vi "Convert Assert Event Data to Test Case - Error - Stack Trace.vi"() -> ()   [LabVIEW 2013, in "JUnit Conversion Tests.lvlib"]
uses:
  JUnit Conversion Tests.lvlib
  <vilib>/addons/_JKI Toolkits/Caraya/classes/Test Result/Assert Event Data (Extended).ctl
  JUnit XML/Test Case/Test Case.lvclass/Test Case.ctl
  JUnit XML/Test Case/Read Stack Trace.vi
  <vilib>/addons/_JKI Toolkits/Caraya/classes/Assert/Assert Equal Value_Variant.vi
  JUnit Conversion/JUnit Conversion.lvlib
  <vilib>/addons/_JKI Toolkits/Caraya/classes/Test Result/Test Result.lvclass
  <vilib>/addons/_JKI Toolkits/Caraya/classes/Assert/Assert.lvclass
  <vilib>/addons/_JKI Toolkits/Caraya/classes/Test/Test.lvclass
  JUnit XML/Test Case/Test Case.lvclass
panel:
  out "error out":errorcluster
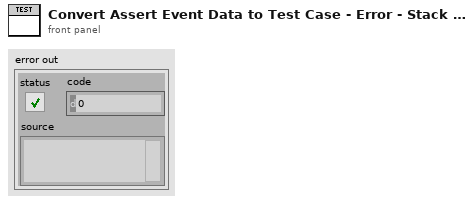
[diagram p1: front panel]
types:
  T1 = typedef "Caraya.lvlib/Test Result.lvclass/Assert Event Data (Extended).ctl" = cluster{"name":string, "passed":bool, "call-chain":string[], "test-error":errorcluster, "timestamp":timestamp, "assert-id":string, "test-id":string, "time":dbl, "message":string, "properties":variant, "measurements":variant, "user-defined":variant}
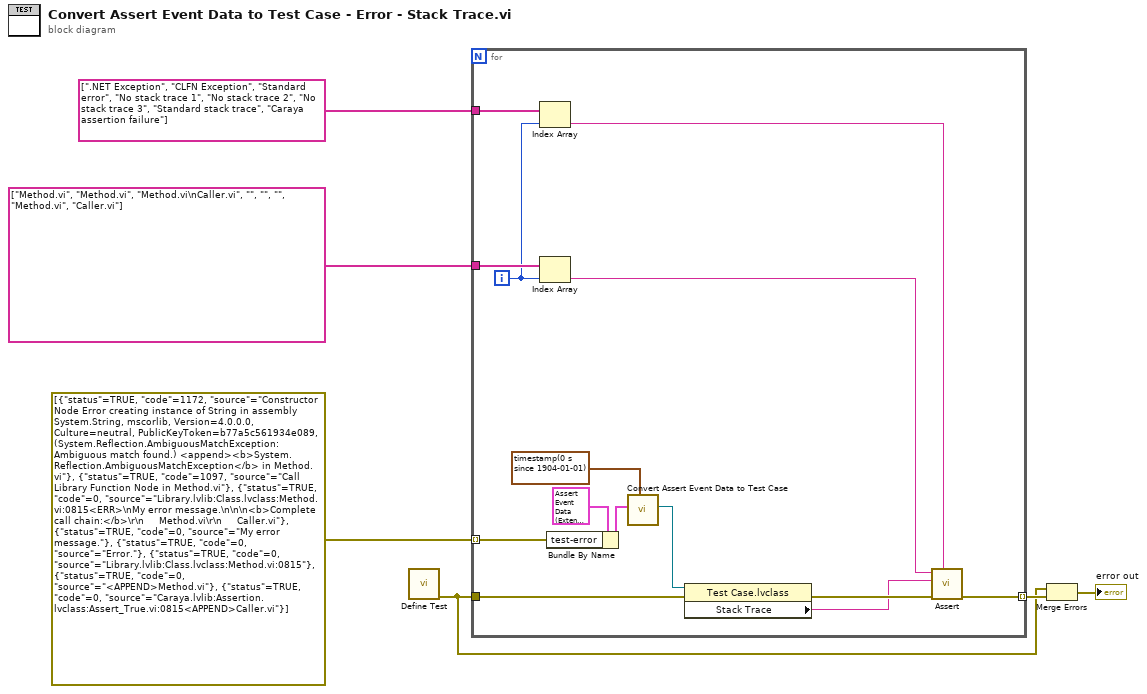
[diagram p0: block diagram]
diagram:
  n1 = call <vilib>:"Define Test.vi"() -> ("error out"=w4:errorcluster)  [unwired: 10 in, 1 out]
  n2 = for {
    tunnel: [w20] -> w6 mode=indexing
    tunnel: w4 -> [w19]
    tunnel: string[] ["Method.vi", "Method.vi", "Method.vi\nCaller.vi", "", "", "", "Method.vi", "Caller.vi"] -> [w13]
    tunnel: errorcluster[] [{"status"=TRUE, "code"=1172, "source"="Constructor Node Error creating instance of String in assembly System.String, mscorlib, Version=4.0.0.0, Culture=neutral, PublicKeyToken=b77a5c561934e089, (System.Reflection.AmbiguousMatchException: Ambiguous match found.) <append><b>System.Reflection.AmbiguousMatchException</b> in Method.vi"}, {"status"=TRUE, "code"=1097, "source"="Call Library Function Node in Method.vi"}, {"status"=TRUE, "code"=0, "source"="Library.lvlib:Class.lvclass:Method.vi:0815<ERR>\nMy error message.\n\n\n<b>Complete call chain:</b>\r\n     Method.vi\r\n     Caller.vi"}, {"status"=TRUE, "code"=0, "source"="My error message."}, {"status"=TRUE, "code"=0, "source"="Error."}, {"status"=TRUE, "code"=0, "source"="Library.lvlib:Class.lvclass:Method.vi:0815"}, {"status"=TRUE, "code"=0, "source"="<APPEND>Method.vi"}, {"status"=TRUE, "code"=0, "source"="Caraya.lvlib:Assertion.lvclass:Assert_True.vi:0815<APPEND>Caller.vi"}] -> [w12] mode=indexing
    tunnel: string[] [".NET Exception", "CLFN Exception", "Standard error", "No stack trace 1", "No stack trace 2", "No stack trace 3", "Standard stack trace", "Caraya assertion failure"] -> [w11]
    i -> [w9]
    n3 = Index Array(array=w11, index=w9) -> (element=w10:string)
    n4 = Index Array(array=w13, index=w9) -> (element=w8:string)
    n5 = Bundle By Name(cluster=T1 {"name"="", "passed"=FALSE, "call-chain"=[], "test-error"={"status"=FALSE, "code"=0, "source"=""}, "timestamp"=timestamp(0 s since 1904-01-01), "assert-id"="", "test-id"="", "time"=-1.0, "message"="", "properties"=variant, "measurements"=variant, "user-defined"=variant} ("Assert Event Data"), "test-error"=w12) -> (w17:T1)
    n6 = call "Convert Assert Event Data to Test Case.vi"("Start Time"=timestamp(0 s since 1904-01-01), "Assert Event Data"=w17) -> ("Test Case"=w16:refnum<class "Test Case.lvclass">)  [unwired: 9 in]
    n7 = property on="Property Node" class="Test Case.lvclass"(reference=w16, error in=w19) -> (error out=w15:errorcluster, "Stack Trace"=w7:string)  [unwired: 1 out]
    n8 = call-poly <vilib>:"Assert.vi"("Label"=w10, "error in (no error)"=w15, "Y"=w7, "X"=w8) -> ("error out"=w20:errorcluster)  [unwired: 6 in, 1 out]
  }
  n9 = Merge Errors(w4, w6) -> (→"error out":errorcluster)
